vi "GetOutputWireBranches.vi"(6 "error in":errorcluster, 9 "Loop in":refnum<class "Loop.lvclass">) -> (0 "error out":errorcluster, 3 "Loop out":refnum<class "Loop.lvclass">, 4 "branches":string[](array[string]))   [LabVIEW 2014, in "Raspberry Pi Compatible Compiler for LabVIEW.lvlib" / "Loop.lvclass"]
uses:
  Loop.lvclass
  Loop.lvclass/Loop.ctl
  ShiftRegister/ShiftRegister.lvclass/ShiftRegister.ctl
  Structure/Structure.lvclass
  RightShiftRegister/RightShiftRegister.lvclass
  ShiftRegister/ShiftRegister.lvclass
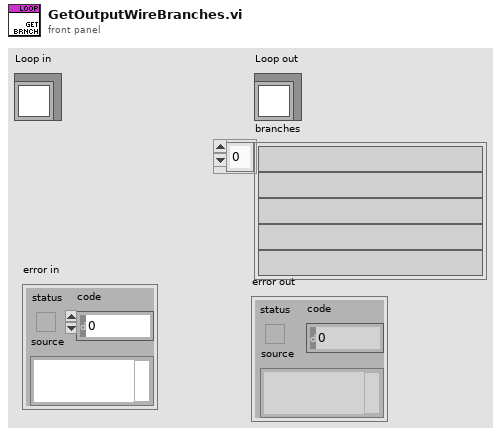
[diagram p1: front panel]
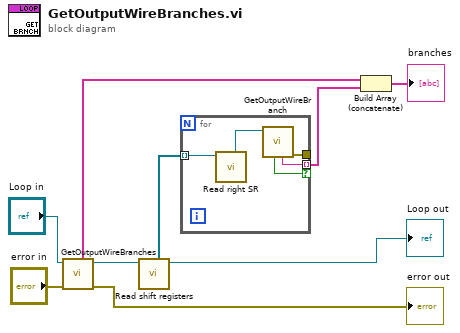
[diagram p0: block diagram]
diagram:
  n1 = call-parent "GetOutputWireBranches.vi"("error in"="error in", "Structure in"="Loop in") -> ("error out"=→"error out":errorcluster, "Structure out"=w7:refnum<class "Loop.lvclass">, "branches"=w2:string[])  [unwired: 5 in]
  n2 = call "Read shift registers.vi"("Loop in"=w7) -> ("Loop out"=→"Loop out":refnum<class "Loop.lvclass">, "shift registers"=w6:refnum<class "ShiftRegister.lvclass">[])  [unwired: 7 in]
  n3 = for {
    tunnel: w6 -> [w14] mode=indexing
    tunnel: [w12] -> w3 mode=indexing if=w11
    tunnel: [w10] -> _
    n4 = call "Read right SR.vi"("ShiftRegister in"=w14) -> ("right SR"=w13:refnum<class "RightShiftRegister.lvclass">)  [unwired: 7 in, 1 out]
    n5 = call-dynamic "GetOutputWireBranch.vi"("Tunnel in"=w13) -> ("error out"=w10:errorcluster, "branches"=w12:string, "branched"=w11:bool)  [unwired: 5 in, 1 out]
  }
  n6 = Build Array (concatenate)(w2, w3) -> (→"branches":string[])
